vi "Run Tests (Project).vi"(10 "Virtual Folder (empty: \"My Computer\")":string, 11 "Project":refnum<vi>) -> (0 "error out":errorcluster)   [LabVIEW 2020, in "Caraya.lvlib"]
uses:
  Caraya.lvlib
  classes/Test Runner/Test Runner.lvclass/Test Runner.ctl
  classes/Test Runner.Project/Test Runner.Project.lvclass
  C:/projects/caraya/src/classes/Test Runner/Test Runner.lvclass
  classes/Test Runner/Test Runner.lvclass
panel:
  # "CARAYA Run Active Project's Unit Tests\n\nThis tool will run all Caraya Unit Tests found in the active project."
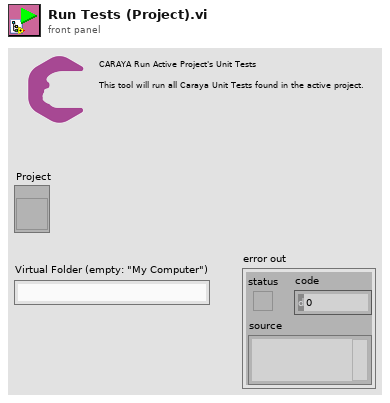
[diagram p1: front panel]
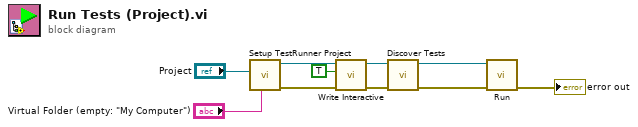
[diagram p0: block diagram]
diagram:
  n1 = call "Setup TestRunner Project.vi"("Virtual Folder (empty: \"My Computer\")"="Virtual Folder (empty: \"My Computer\")", "Project Refnum"="Project") -> ("error out"=w9:errorcluster, "Test Runner.Project out"=w7:refnum<class "Test Runner.Project.lvclass">)  [unwired: 8 in]
  n2 = call "Write Interactive.vi"("Interactive"=TRUE, "Test Runner in"=w7) -> ("Test Runner out"=w6:refnum<class "Test Runner.Project.lvclass">)  [unwired: 9 in]
  n3 = call "Discover Tests.vi"("error in (no error)"=w9, "Test Runner in"=w6) -> ("error out"=w3:errorcluster, "Test Runner out"=w4:refnum<class "Test Runner.Project.lvclass">)  [unwired: 8 in]
  n4 = call "Run.vi"("error in (no error)"=w3, "Test Runner in"=w4) -> ("error out"=→"error out":errorcluster)  [unwired: 7 in, 2 out]
